vi "读取开始时间.vi"(8 "error in (no error)":errorcluster caption="错误输入（无错误）", 11 "定时器类输入":refnum<class "定时器类.lvclass">) -> (0 "error out":errorcluster caption="错误输出", 2 "开始时间":u32, 3 "定时器类输出":refnum<class "定时器类.lvclass">)   [LabVIEW 2014, in "定时器类.lvclass"]
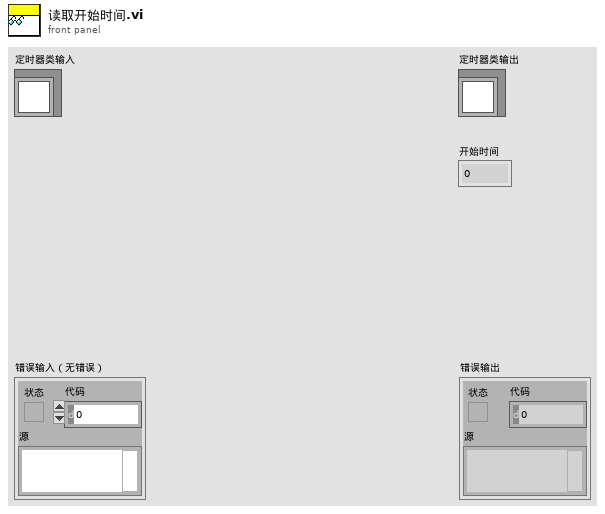
[diagram p1: front panel]
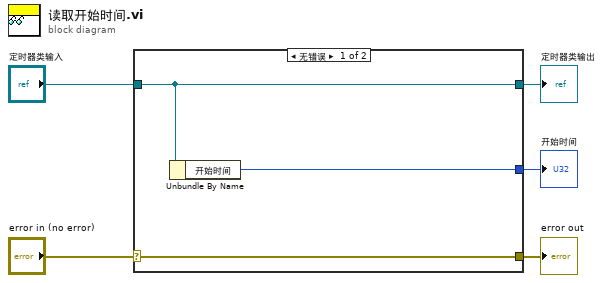
[diagram p0: block diagram]
diagram:
  n1 = case shown="无错误" "error in (no error)" {
    selector: "error in (no error)" -> [w8 w9]
    tunnel: [w8 w9] -> w4
    tunnel: [w7 w10] -> w2
    tunnel: "定时器类输入" -> [w7 w10]
    tunnel: [w6 _] -> w1
    frame No Error {
      n2 = Unbundle By Name(w7) -> ("开始时间"=w6:u32)
    }
    frame Error {
    }
  }
  "error out" <- w4
  "定时器类输出" <- w2
  "开始时间" <- w1
